vi "Update Task State.vi"(7 "State":T1, 8 "error in (no error)":errorcluster, 11 "Task in":refnum<class "Task.lvclass">) -> (0 "error out":errorcluster, 3 "Task out":refnum<class "Task.lvclass">)   [LabVIEW 2020, in "Volatus.lvlib" / "Task.lvclass"]
uses:
  Task.lvclass
  C:/Program Files (x86)/National Instruments/LabVIEW 2020/vi.lib/ActorFramework/Actor/Actor.lvclass
  Task State.ctl
  Task.lvclass/Task.ctl
  <vilib>/ActorFramework/Actor/Actor.lvclass/Actor.ctl
  TaskStateHandler Messages/Update Nested State Msg/Update Nested State Msg.lvclass/Update Nested State Msg.ctl
  <vilib>/ActorFramework/Message Enqueuer/Message Enqueuer.lvclass/Message Enqueuer.ctl
  Event API/EventAPI.lvclass/EventAPI.ctl
  EventHandler Messages/Handle Event Msg/Handle Event Msg.lvclass/Handle Event Msg.ctl
  <vilib>/ActorFramework/Message Enqueuer/Enqueue.vi
  Report Event.vi
  Event API/Report Event.vi
  EventHandler Messages/Handle Event Msg/Send Handle Event.vi
  TaskStateHandler Messages/Update Nested State Msg/Update Nested State Msg.lvclass
  C:/Program Files (x86)/National Instruments/LabVIEW 2020/vi.lib/ActorFramework/Message/Message.lvclass
  EventHandler Messages/Handle Event Msg/Handle Event Msg.lvclass
  <vilib>/ActorFramework/Message Priority Queue/Priority Enqueue.vi
  <vilib>/Utility/LVClass/Get LV Class Name.vi
  <vilib>/ActorFramework/Message Enqueuer/Message Enqueuer.lvclass
  <vilib>/ActorFramework/Actor/Actor.lvclass
  Volatus.lvlib
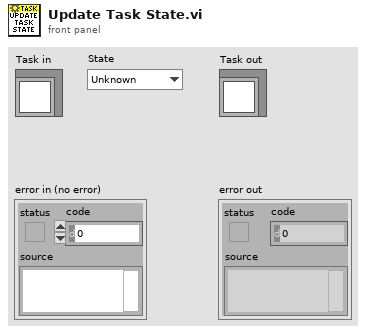
[diagram p1: front panel]
types:
  T1 = typedef "Volatus.lvlib/Task State.ctl" = enum16{"Unknown", "Idle", "Initializing", "Starting", "Running", "Stopping", "Stopped", "Error - Init", "Error - Start", "Error - Run", "Error - Stop"}
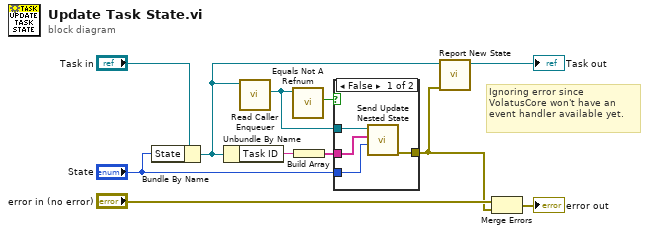
[diagram p0: block diagram]
diagram:
  # "Ignoring error since VolatusCore won't have an event handler available yet."
  n1 = Bundle By Name(cluster="Task in", "State"="State") -> (w3:refnum<class "Task.lvclass">)
  n2 = Unbundle By Name(w3) -> ("Task ID"=w10:string)
  n3 = call <vilib>:"Read Caller Enqueuer.vi"("Actor"=w3) -> ("Caller Enqueuer"=w5:refnum<class "Message Enqueuer.lvclass">)  [unwired: 10 in]
  n4 = call <vilib>:"Equals Not A Refnum.vi"("Message Enqueuer"=w5) -> ("Not a refnum?"=w4:bool)  [unwired: 10 in]
  n5 = Build Array(w10) -> (w9:string[])
  n6 = case shown="False" w4 {
    tunnel: w9 -> [w15 _]
    tunnel: "State" -> [w14 _]
    tunnel: [w13 _] -> w1
    tunnel: w5 -> [w12 _]
    frame False {
      n7 = call "Send Update Nested State.vi"("State"=w14, "Task Hierarchy"=w15, "Message Enqueuer"=w12) -> ("error out"=w13:errorcluster)  [unwired: 7 in, 1 out]
    }
    frame True {
    }
  }
  n8 = call "Report New State.vi"("error in (no error)"=w1, "Task in"=w3) -> ("Task out"=→"Task out":refnum<class "Task.lvclass">)  [unwired: 8 in, 1 out]
  n9 = Merge Errors("error in (no error)", w1) -> (→"error out":errorcluster)
